vi "niRFUtil MEAS Max and Min (complex array).vi"(2 "Complex Array In":cdb[](array[numeric]) format="%.2f") -> (6 "Max":csg format="%.2f", 7 "Min":csg format="%.2f")   [LabVIEW 2015, in "niRFUtil.lvlib"]
doc: "(c) Copyright 2006, National Instruments, Inc. This VI may not be duplicated, sold, or distributed without written consent from National Instruments."
uses:
  niRFUtil.lvlib
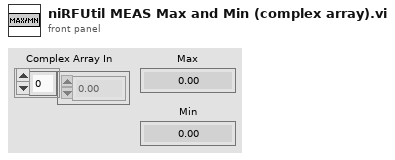
[diagram p1: front panel]
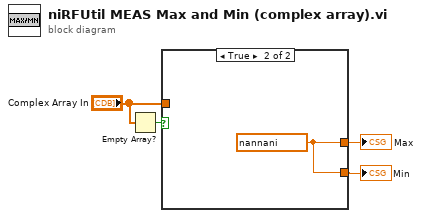
[diagram p0: block diagram]
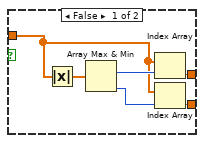
[diagram p2: hidden frame]
diagram:
  n1 = Empty Array?(array="Complex Array In") -> (empty?=w2:bool)
  n2 = case shown="True" w2 {
    tunnel: "Complex Array In" -> [w7 _]
    tunnel: [w6 w11] -> w4
    tunnel: [w5 w11] -> w3
    frame False {
      n3 = Absolute Value(x=w7) -> (abs(x)=w10:dbl[])
      n4 = Array Max & Min(array=w10) -> (max index (indices)=w9:i32, min index (indices)=w8:i32)  [unwired: 2 out]
      n5 = Index Array(array=w7, index=w9) -> (element=w5:cdb)
      n6 = Index Array(array=w7, index=w8) -> (element=w6:cdb)
    }
    frame True {
      w11 = cdb nan+nani ("Signal")
    }
  }
  "Max" <- w3
  "Min" <- w4
